vi "SNAFU to Decimal.vi"(11 "SNAFU":string) -> (3 "Decimal":i64)   [LabVIEW 2021, in "d25.lvlib"]
uses:
  d25.lvlib
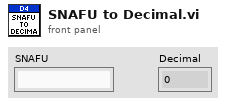
[diagram p1: front panel]
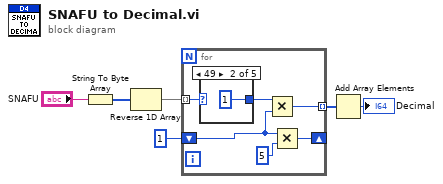
[diagram p0: block diagram]
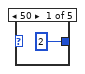
[diagram p2: hidden frame]
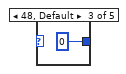
[diagram p3: hidden frame]
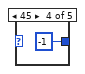
[diagram p4: hidden frame]
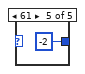
[diagram p5: hidden frame]
diagram:
  n1 = String To Byte Array(string="SNAFU") -> (unsigned byte array=w3:u8[])
  n2 = Reverse 1D Array(array=w3) -> (reversed array=w2:u8[])
  n3 = for {
    tunnel: w2 -> [w12] mode=indexing
    tunnel: [w10] -> w5 mode=indexing
    shift-right: [w8] -> _
    shift-left: i64 1 ("y") -> [w9]
    n4 = case shown="49" w12 {
      tunnel: [i64 2 i64 1 i64 0 i64 -1 i64 -2] -> w11
      frame 50 {
        # "2"
      }
      frame 49 {
        # "2"
      }
      frame 48, Default {
        # "2"
      }
      frame 45 {
        # "2"
      }
      frame 61 {
        # "2"
      }
    }
    n5 = Multiply(x=w11, y=w9) -> (x*y=w10:i64)
    n6 = Multiply(x=w9, y=i64 5) -> (x*y=w8:i64)
  }
  n7 = Add Array Elements(numeric array=w5) -> (sum=→"Decimal":i64)
